vi "Helmholtz2D_Cal Coef Mtrx_Dirichlet.vi"(9 "Domain":T2={"x"={"start x"=0.0, "end x"=1.0, "# of x-points"=11}, "y"={"start y"=0.0, "end y"=1.0, "# of y-points"=11}}, 10 "a":dbl, 11 "k":dbl=1.0) -> (2 "D":T1, 3 "C":T1)   [LabVIEW 2020, in "NI_PDE.lvlib"]
uses:
  <vilib>/gmath/NI_PDE.lvlib
  <vilib>/Analysis/Matrix/Datatypes/RealMatrix.ctl
  <vilib>/Analysis/7linalg.llb/Create Special Real Matrix.vi
  <vilib>/Analysis/Matrix/Numeric/Multiply/Multiply - R,RM.vi
  <vilib>/Analysis/Matrix/Numeric/Add/Add - RM,RM.vi
  <vilib>/Analysis/Matrix/Numeric/Multiply/Multiply - RM,R.vi
  <vilib>/Analysis/NI_AALPro.lvlib
  <vilib>/Analysis/Matrix/NI_Matrix.lvlib
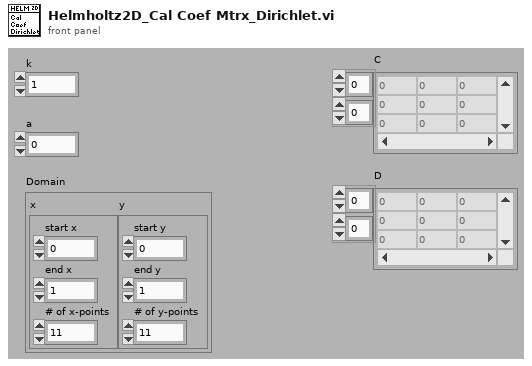
[diagram p1: front panel]
types:
  T1 = typedef "NI_Matrix.lvlib/RealMatrix.ctl" = dbl[][]
  T2 = cluster{"x":cluster{"start x":dbl, "end x":dbl, "# of x-points":i32}, "y":cluster{"start y":dbl, "end y":dbl, "# of y-points":i32}}
  T3 = enum32{"Identity", "Diagonal", "Toepliz", "Vandermonde", "Companion"}
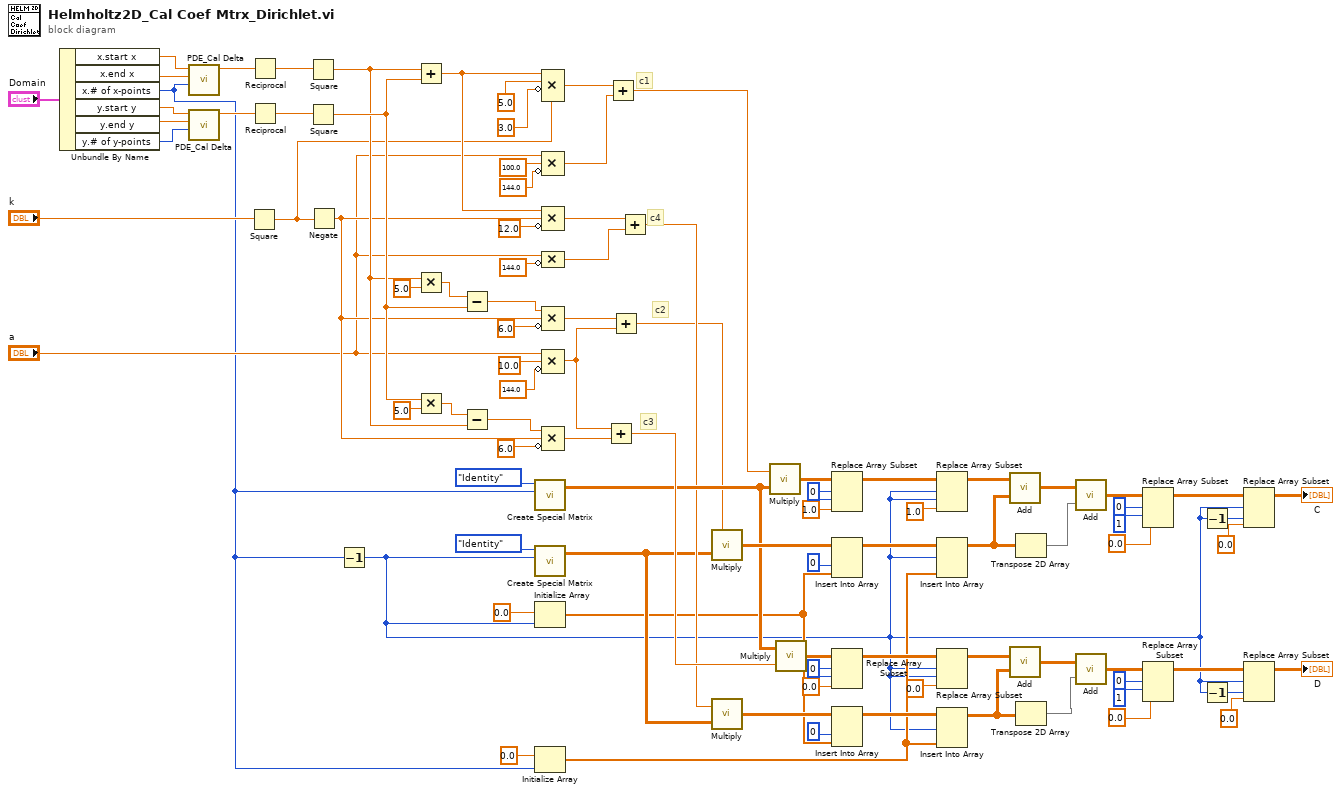
[diagram p0: block diagram]
diagram:
  w35 = 0 ("index (row)")
  w75 = 0 ("index (row)")
  # "c3"
  # "c2"
  # "c4"
  # "c1"
  n1 = Unbundle By Name("Domain") -> ("x.start x"=w94:dbl, "x.end x"=w93:dbl, "x.# of x-points"=w5:i32, "y.start y"=w91:dbl, "y.end y"=w92:dbl, "y.# of y-points"=w90:i32)
  n2 = call <vilib>:"PDE_Cal Delta.vi"("# of points"=w5, "end"=w93, "start"=w94) -> ("delta"=w7:dbl)  [unwired: 8 out]
  n3 = call <vilib>:"PDE_Cal Delta.vi"("# of points"=w90, "end"=w92, "start"=w91) -> ("delta"=w6:dbl)  [unwired: 8 out]
  n4 = Square(x="k") -> (x^2=w1:dbl)
  n5 = Reciprocal(x=w7) -> (1/x=w3:dbl)
  n6 = Reciprocal(x=w6) -> (1/x=w2:dbl)
  n7 = Square(x=w3) -> (x^2=w41:dbl)
  n8 = Square(x=w2) -> (x^2=w42:dbl)
  n9 = Negate(x=w1) -> (-x=w39:dbl)
  n10 = Decrement(x=w5) -> (x-1=w4:i32)
  n11 = Add(x=w41, y=w42) -> (x+y=w59:dbl)
  n12 = Multiply(x=w41, y=5.0) -> (x*y=w53:dbl)
  n13 = Multiply(x=w42, y=5.0) -> (x*y=w44:dbl)
  n14 = Subtract(x=w53, y=w42) -> (x-y=w52:dbl)
  n15 = Subtract(x=w44, y=w41) -> (x-y=w45:dbl)
  n16 = call-poly <vilib>:"Create Special Matrix.vi"("matrix type"=T3."Identity", "matrix size"=w5) -> ("Special Matrix"=w36:T1)  [unwired: 2 in, 2 out]
  n17 = call-poly <vilib>:"Create Special Matrix.vi"("matrix type"=T3."Identity", "matrix size"=w4) -> ("Special Matrix"=w28:T1)  [unwired: 2 in, 2 out]
  n18 = Initialize Array(0.0 ("element"), w4) -> (w24:dbl[])
  n19 = Initialize Array(0.0 ("element"), w5) -> (w22:dbl[])
  n20 = Compound Arithmetic op=MULTIPLY(w59, 5.0 ("y"), invert 3.0 ("y"), w1) -> (w65:dbl)
  n21 = Compound Arithmetic op=MULTIPLY("a", 100.0 ("y"), invert 144.0 ("y")) -> (w62:dbl)
  n22 = Compound Arithmetic op=MULTIPLY(w59, w39, invert 12.0 ("y")) -> (w57:dbl)
  n23 = Compound Arithmetic op=MULTIPLY("a", invert 144.0 ("y")) -> (w55:dbl)
  n24 = Compound Arithmetic op=MULTIPLY(w52, w39, invert 6.0 ("y")) -> (w50:dbl)
  n25 = Compound Arithmetic op=MULTIPLY("a", 10.0 ("y"), invert 144.0 ("y")) -> (w38:dbl)
  n26 = Compound Arithmetic op=MULTIPLY(w45, w39, invert 6.0 ("y")) -> (w47:dbl)
  n27 = Add(x=w38, y=w47) -> (x+y=w37:dbl)
  n28 = Add(x=w65, y=w62) -> (x+y=w40:dbl)
  n29 = Add(x=w50, y=w38) -> (x+y=w27:dbl)
  n30 = Add(x=w57, y=w55) -> (x+y=w29:dbl)
  n31 = call-poly <vilib>:"Multiply.vi"("Real Matrix A"=w28, "Real Scalar c"=w27) -> ("c * A"=w85:T1)
  n32 = call-poly <vilib>:"Multiply.vi"("Real Matrix A"=w28, "Real Scalar c"=w29) -> ("c * A"=w26:T1)
  n33 = call-poly <vilib>:"Multiply.vi"("Real Matrix A"=w36, "Real Scalar c"=w40) -> ("c * A"=w74:T1)
  n34 = call-poly <vilib>:"Multiply.vi"("Real Scalar c"=w37, "Real Matrix A"=w36) -> ("A * c"=w31:T1)
  n35 = Replace Array Subset(array=w74, new element=1.0 ("new element/subarray"), index (row)=w75, index (col)=w75) -> (w77:T1)
  n36 = Insert Into Array(array=w85, index (col)=0 ("disabled index (col)"), new element=w24) -> (w83:T1)  [unwired: 1 in]
  n37 = Replace Array Subset(array=w31, new element=0.0 ("new element/subarray"), index (row)=w35, index (col)=w35) -> (w33:T1)
  n38 = Insert Into Array(array=w26, index (col)=0 ("disabled index (col)"), new element=w24) -> (w23:T1)  [unwired: 1 in]
  n39 = Replace Array Subset(array=w77, new element=1.0 ("new element/subarray"), index (row)=w4, index (col)=w4) -> (w73:T1)
  n40 = Insert Into Array(array=w83, index (row)=w4, new element=w22) -> (w81:T1)  [unwired: 1 in]
  n41 = Replace Array Subset(array=w33, new element=0.0 ("new element/subarray"), index (row)=w4, index (col)=w4) -> (w30:T1)
  n42 = Insert Into Array(array=w23, index (row)=w4, new element=w22) -> (w21:T1)  [unwired: 1 in]
  n43 = call-poly <vilib>:"Add.vi"("Real Matrix B"=w81, "Real Matrix A"=w73) -> ("A + B"=w80:T1)
  n44 = call-poly <vilib>:"Add.vi"("Real Matrix B"=w21, "Real Matrix A"=w30) -> ("A + B"=w20:T1)
  n45 = Transpose 2D Array(2D array=w81) -> (transposed array=w79:T1)
  n46 = Transpose 2D Array(2D array=w21) -> (transposed array=w19:T1)
  n47 = call-poly <vilib>:"Add.vi"("Real Matrix B"=w79, "Real Matrix A"=w80) -> ("A + B"=w69:T1)
  n48 = call-poly <vilib>:"Add.vi"("Real Matrix B"=w19, "Real Matrix A"=w20) -> ("A + B"=w12:T1)
  n49 = Replace Array Subset(array=w69, new element=0.0 ("new element/subarray"), index (row)=0, index (col)=1 ("index (row)")) -> (w72:T1)
  n50 = Replace Array Subset(array=w12, new element=0.0 ("new element/subarray"), index (row)=0, index (col)=1 ("index (row)")) -> (w13:T1)
  n51 = Decrement(x=w4) -> (x-1=w66:i32)
  n52 = Decrement(x=w4) -> (x-1=w18:i32)
  n53 = Replace Array Subset(array=w72, new element=0.0 ("new element/subarray"), index (row)=w4, index (col)=w66) -> (→"C":T1)
  n54 = Replace Array Subset(array=w13, new element=0.0 ("new element/subarray"), index (row)=w4, index (col)=w18) -> (→"D":T1)
